vi "waitOnIRQ.vi"(8 "error in (no error)":errorcluster, 10 "Timeout":i32, 11 "ModbusIRQ in":refnum<class "ModbusIRQ.lvclass">) -> (0 "error out":errorcluster, 1 "TimedOut":bool, 2 "IRQs":i32[](array[numeric]), 3 "ModbusIRQ out":refnum<class "ModbusIRQ.lvclass">)   [LabVIEW 2016, in "ModbusIRQ.lvclass"]
uses:
  ModbusIRQ.lvclass
  ModbusIRQ.lvclass/ModbusIRQ.ctl
  FPGA/FPGA.lvclass
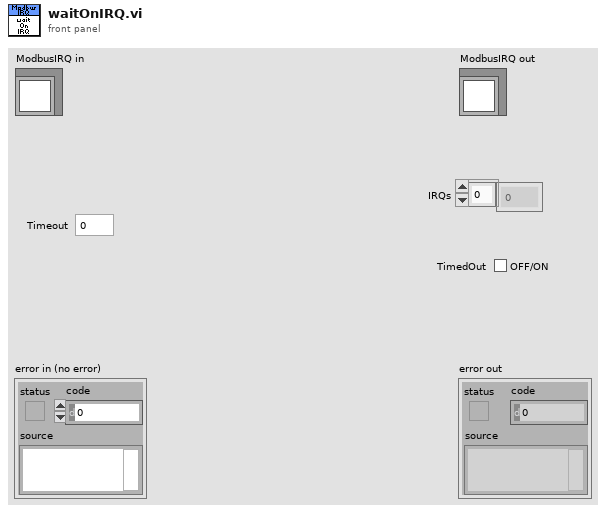
[diagram p1: front panel]
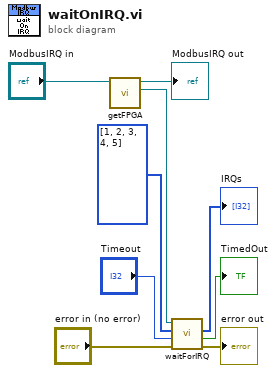
[diagram p0: block diagram]
diagram:
  n1 = call "getFPGA.vi"("ModbusIRQ in"="ModbusIRQ in") -> ("FPGA"=w9:refnum<class "FPGA.lvclass">, "ModbusIRQ out"=→"ModbusIRQ out":refnum<class "ModbusIRQ.lvclass">)  [unwired: 9 in]
  n2 = call "waitForIRQ.vi"("error in (no error)"="error in (no error)", "Timeout (ms)"="Timeout", "IRQs in"=i32[] [1, 2, 3, 4, 5], "FPGA in"=w9) -> ("error out"=→"error out":errorcluster, "TimedOut"=→"TimedOut":bool, "IRQs out"=→"IRQs":i32[])  [unwired: 4 in, 1 out]
